vi "Get Sensor Params by Index.vi"(9 "index":i32) -> (3 "Sensor Cfg Params":T1 {"CalibrCoefArray" format="%#.12g"})   [LabVIEW 2015, in "Tool Cfg.lvlib"]
uses:
  Tool Cfg.lvlib
  _SensorConfigParams Cluster--typedef.ctl
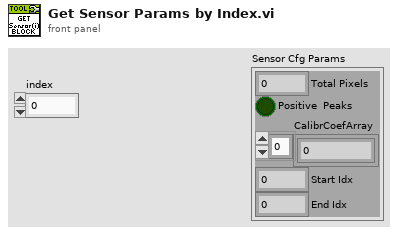
[diagram p1: front panel]
types:
  T1 = typedef "Tool Cfg.lvlib/_SensorConfigParams Cluster--typedef.ctl" = cluster{"Total Pixels":u16, "Positive  Peaks":bool, "CalibrCoefArray":dbl[], "Start Idx":u16, "End Idx":u16}
  T2 = typedef "Tool Cfg.lvlib/_Sensor Block Cluster--typedef.ctl" = cluster{"nSensors":u16, "SensorCfgParams Array":T1[]}
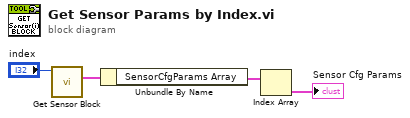
[diagram p0: block diagram]
diagram:
  n1 = call "Get Sensor Block.vi"("Select Probe"="index") -> ("Sensor Block"=w3:T2)  [unwired: 10 in]
  n2 = Unbundle By Name(w3) -> ("SensorCfgParams Array"=w2:T1[])
  n3 = Index Array(array=w2) -> (element=→"Sensor Cfg Params":T1)  [unwired: 1 in]
